vi "variabel retarder.vi"(5 "Stop":bool, 8 "Error in":errorcluster) -> (0 "Error Out":errorcluster)   [LabVIEW 2018]
uses:
  <vilib>/DAQmx/write.llb/DAQmx Write (Analog 1D Wfm NChan NSamp).vi
  <vilib>/DAQmx/create/channels.llb/DAQmx Create Channel (AO-Voltage-Basic).vi
  <vilib>/DAQmx/configure/timing.llb/DAQmx Timing (Sample Clock).vi
  <vilib>/DAQmx/miscellaneous.llb/DAQmx Fill In Error Info.vi
  <resource>/objmgr/daqmx.rc
  <vilib>/measure/NI_MABase.lvlib
panel:
  out "Waveform Graph":waveform(dbl)[](graph)=[{"t0"=timestamp(0 s since 1904-01-01), "dt"=0.001, "Y"=[]}]
  in  "Output Array":T1(array[cluster])=[{"Waveform Type"=0, "Amplitude"=1.0, "Frequency"=10.0}] {"Frequency" format="%0.2p"; "Amplitude" format="%0.2p"; "Waveform Type" items=["Sine Wave", "Triangle Wave", "Square Wave", "Sawtooth Wave"]}
  in  "Number of Samples":i32=500
  in  "Sample Rate":dbl=1000000.0
  in  "Sample Clock Source":tag="OnboardClock"
  in  "Max Voltage":dbl=1.841
  in  "Min Voltage":dbl=-1.841
  in  "Physical Channel(s)":tag="GalvoCtrl/ao2"
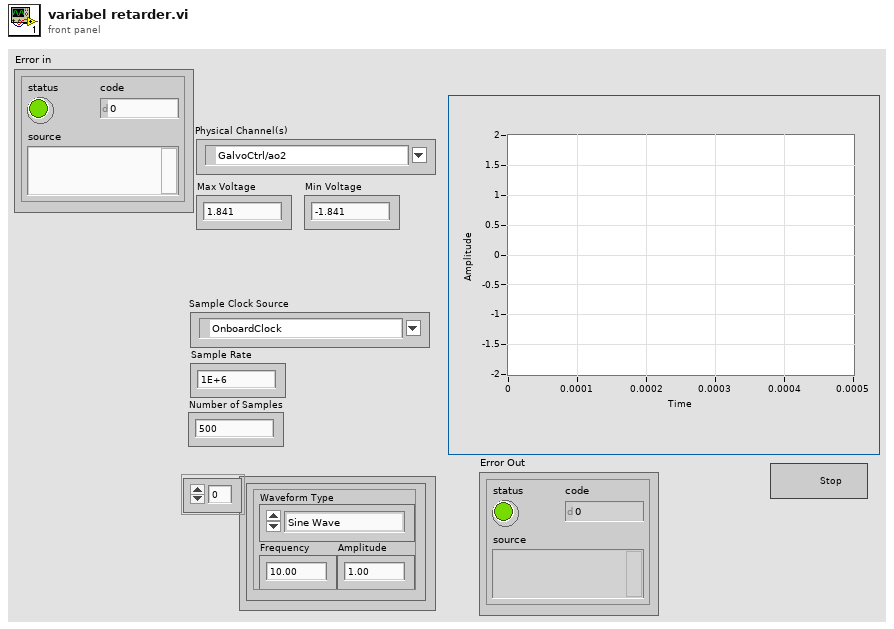
[diagram p1: front panel]
types:
  T1 = cluster{"Waveform Type":u16, "Amplitude":dbl, "Frequency":dbl}[]
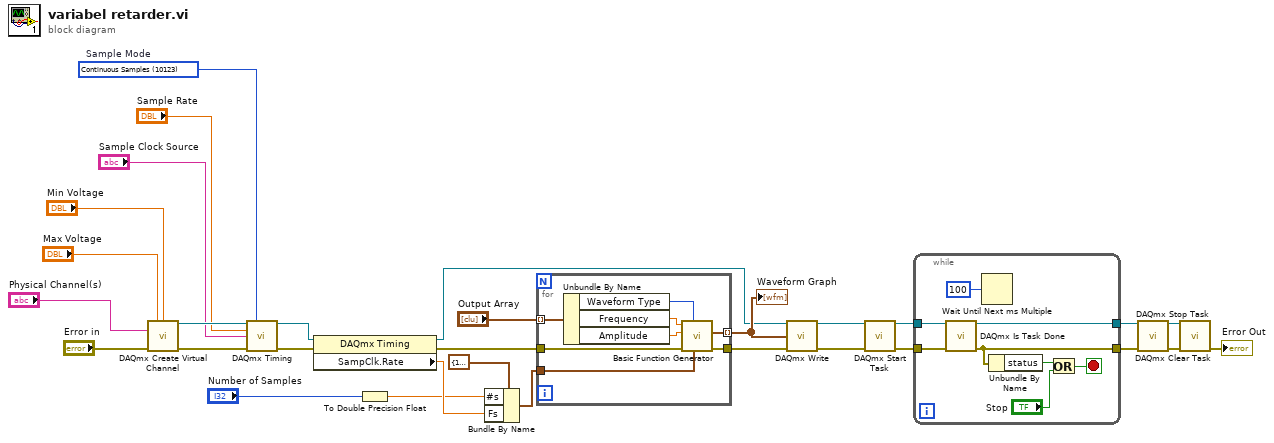
[diagram p0: block diagram]
diagram:
  w28 = 10123 items=["Finite Samples"=10178, "Continuous Samples"=10123, "Hardware Timed Single Point"=12522]  # Sample Mode
  n1 = call-poly <vilib>:"DAQmx Create Virtual Channel.vi"("maximum value"="Max Voltage", "minimum value"="Min Voltage", "physical channels"="Physical Channel(s)", "error in"="Error in") -> ("task out"=w26:refnum<k21>, "error out"=w27:errorcluster)  [unwired: 10 in]
  n2 = call-poly <vilib>:"DAQmx Timing.vi"("task/channels in"=w26, "sample mode"=w28, "rate"="Sample Rate", "source"="Sample Clock Source", "error in"=w27) -> ("task out"=w30:refnum<k21>, "error out"=w29:errorcluster)  [unwired: 9 in]
  n3 = property class="DAQmx Timing"(reference=w30, error in=w29) -> (reference out=w3:refnum<k21>, error out=w4:errorcluster, "SampClk.Rate"=w17:dbl)
  n4 = To Double Precision Float(number="Number of Samples") -> (double precision float=w10:dbl)
  n5 = Bundle By Name(cluster=cluster{"Fs":dbl, "#s":dbl} {"Fs"=1000.0, "#s"=1000.0} ("sampling info"), "#s"=w10, "Fs"=w17) -> (w16:cluster{"Fs":dbl, "#s":dbl})
  n6 = for {
    tunnel: w4 -> [w38]
    tunnel: w16 -> [w37]
    tunnel: [w36] -> w13
    tunnel: "Output Array" -> [w35] mode=indexing
    tunnel: [w31] -> w11 mode=indexing
    n7 = Unbundle By Name(w35) -> ("Waveform Type"=w34:u16, "Frequency"=w33:dbl, "Amplitude"=w32:dbl)
    n8 = call <vilib>:"Basic Function Generator.vi"("sampling info"=w37, "signal type"=w34, "error in (no error)"=w38, "amplitude"=w32, "frequency"=w33) -> ("error out"=w36:errorcluster, "signal out"=w31:waveform(dbl))  [unwired: 4 in, 1 out]
  }
  "Waveform Graph" <- w11
  n9 = call-poly <vilib>:"DAQmx Write.vi"("task/channels in"=w3, "data"=w11, "error in"=w13) -> ("task out"=w15:refnum<k21>, "error out"=w14:errorcluster)  [unwired: 10 in, 1 out]
  n10 = call <vilib>:"DAQmx Start Task.vi"("task/channels in"=w15, "error in"=w14) -> ("task out"=w25:refnum<k21>, "error out"=w24:errorcluster)  [unwired: 12 in]
  n11 = while {
    tunnel: w25 -> [w46]
    tunnel: w24 -> [w45]
    tunnel: [w42] -> w5
    tunnel: [w43] -> w6
    stop <- w44 stop-if-true
    n12 = call <vilib>:"DAQmx Is Task Done.vi"("task/channels in"=w46, "error in"=w45) -> ("task out"=w43:refnum<k21>, "error out"=w42:errorcluster)  [unwired: 11 in, 1 out]
    n13 = Wait Until Next ms Multiple(millisecond multiple=u32 100) -> ()  [unwired: 1 out]
    n14 = Unbundle By Name(w42) -> ("status"=w41:bool)
    n15 = Or(x=w41, y="Stop") -> (x .or. y?=w44:bool)
  }
  n16 = call <vilib>:"DAQmx Stop Task.vi"("task/channels in"=w6, "error in"=w5) -> ("task out"=w8:refnum<k21>, "error out"=w7:errorcluster)  [unwired: 12 in]
  n17 = call <vilib>:"DAQmx Clear Task.vi"("task in"=w8, "error in"=w7) -> ("error out"=→"Error Out":errorcluster)  [unwired: 13 in]
